vi "TVC_PAT.vi"() -> ()   [LabVIEW 2019]
uses:
  <vilib>/Utility/error.llb/DialogType.ctl
  <vilib>/DAQmx/read.llb/DAQmx Read (Analog 1D DBL NChan 1Samp).vi
  <vilib>/DAQmx/create/channels.llb/DAQmx Create Channel (AI-Voltage-Basic).vi
  <vilib>/DAQmx/configure/timing.llb/DAQmx Timing (Sample Clock).vi
  <vilib>/DAQmx/miscellaneous.llb/DAQmx Fill In Error Info.vi
panel:
  out "THETA ANGLE":dbl(knob) scale=-45.0..45.0
  out "PHI ANGLE":dbl(knob) scale=-45.0..45.0
  in  "Testing Name":string="Postion Accuracy Test"
  in  "File Path":path=path "C:/Users/Kaylin Gopal/Desktop/TVC_electronics/PAT1.tdms"
  in  "?":bool
  in  "Y-Axis":tag
  in  "X-Axis":tag
  # "Channel Settings"
  # "Team: Thrust Vector Control\nTest: Position Accuracy \nAuthour: Kaylin Gopal\n\nPurpose:\n\nDetermine the vectoring accuraccy of the \nthrust vector control test stand."
  # "Equipment:\n\n1. Ultramotion A2 actuators (P - controller)\n2. TE dual axis inclinometer\n3. TVC test stand"
  # "File Settings"
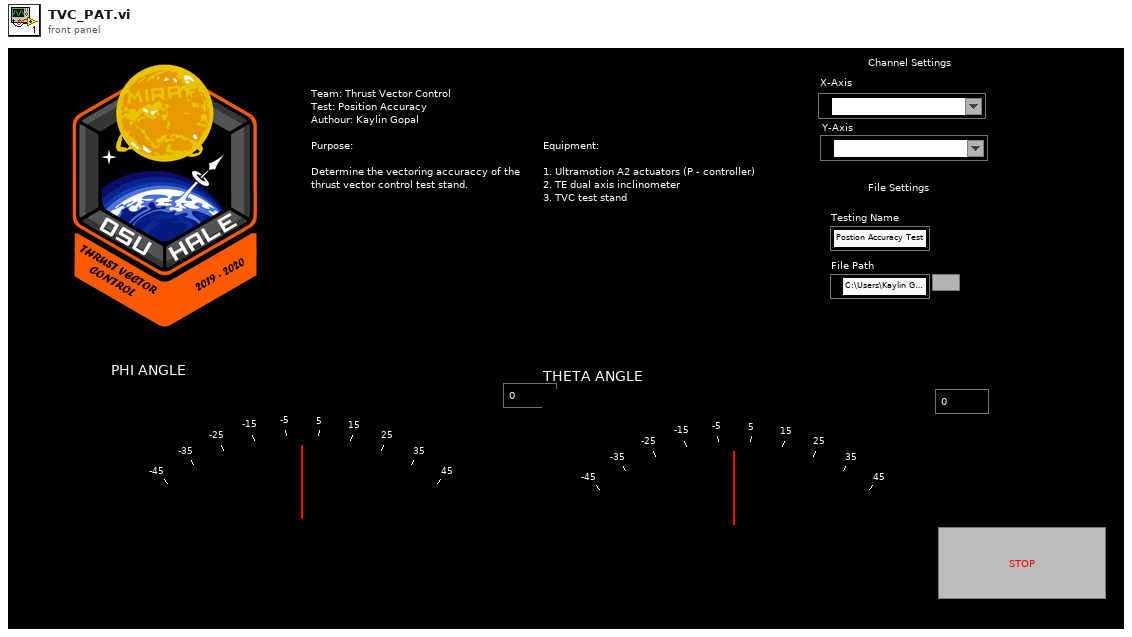
[diagram p1: front panel]
types:
  T1 = typedef "DialogType.ctl" = u16
  T2 = enum16{"open", "open or create", "create or replace", "create", "open (read-only)"}
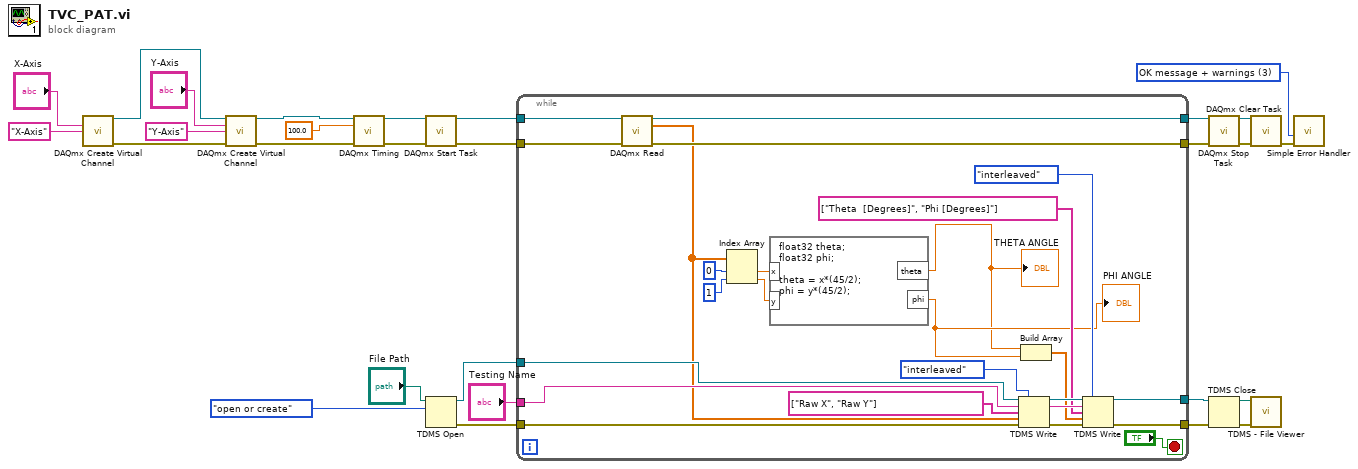
[diagram p0: block diagram]
diagram:
  w3 = T1 3 items=["no dialog", "OK message", "continue or stop message", "OK message + warnings", "continue/stop + warnings"] ("type of dialog (OK msg:1)")
  n1 = call-poly <vilib>:"DAQmx Create Virtual Channel.vi"("physical channels"="X-Axis", "name to assign"="X-Axis") -> ("task out"=w28:refnum<k21>, "error out"=w27:errorcluster)  [unwired: 12 in]
  n2 = call-poly <vilib>:"DAQmx Create Virtual Channel.vi"("task in"=w28, "physical channels"="Y-Axis", "name to assign"="Y-Axis", "error in"=w27) -> ("task out"=w21:refnum<k21>, "error out"=w22:errorcluster)  [unwired: 10 in]
  n3 = call-poly <vilib>:"DAQmx Timing.vi"("task/channels in"=w21, "rate"=100.0, "error in"=w22) -> ("task out"=w18:refnum<k21>, "error out"=w19:errorcluster)  [unwired: 11 in]
  n4 = call <vilib>:"DAQmx Start Task.vi"("task/channels in"=w18, "error in"=w19) -> ("task out"=w16:refnum<k21>, "error out"=w17:errorcluster)  [unwired: 12 in]
  n5 = TDMS Open(10:T2."open or create" ("operation (0:open)"), 11:"File Path") -> (0:w14:errorcluster, 3:w15:refnum<k34>)  [unwired: 5 in]
  n6 = while {
    tunnel: w17 -> [w49]
    tunnel: w16 -> [w48]
    tunnel: w15 -> [w52]
    tunnel: w14 -> [w51]
    tunnel: "Testing Name" -> [w50]
    tunnel: [w40] -> w10
    tunnel: [w39] -> w9
    tunnel: [w45] -> w8
    tunnel: [w44] -> w7
    stop <- "?" stop-if-true
    n7 = call-poly <vilib>:"DAQmx Read.vi"("task/channels in"=w48, "error in"=w49) -> ("task out"=w45:refnum<k21>, "data"=w32:dbl[], "error out"=w44:errorcluster)  [unwired: 11 in]
    n8 = Index Array(array=w32, index #1=0 ("index"), index #2=1 ("index")) -> (element #1=w31:dbl, element #2=w36:dbl)
    n9 = formula code="float32 theta;\nfloat32 phi;\n\ntheta = x*(45/2);\nphi = y*(45/2);"("x"=w31, "y"=w36) -> ("theta"=w29:sgl, "phi"=w30:sgl)
    "THETA ANGLE" <- w29
    "PHI ANGLE" <- w30
    n10 = TDMS Write(0:w52, 1:enum16{"decimated", "interleaved"}."interleaved" ("data layout (0:decimated)"), 5:w50, 7:string[] ["Raw X", "Raw Y"] ("channel name(s) in (Untitled)"), 9:w32, 11:w51) -> (4:w43:refnum<k34>, 6:w41:string, 15:w42:errorcluster)  [unwired: 1 out]
    n11 = Build Array(w29, w30) -> (w34:sgl[])
    n12 = TDMS Write(0:w43, 1:enum16{"decimated", "interleaved"}."interleaved" ("data layout (0:decimated)"), 5:w41, 7:string[] ["Theta  [Degrees]", "Phi [Degrees]"] ("channel name(s) in (Untitled)"), 9:w34, 11:w42) -> (4:w40:refnum<k34>, 15:w39:errorcluster)  [unwired: 2 out]
  }
  n13 = call <vilib>:"DAQmx Stop Task.vi"("task/channels in"=w8, "error in"=w7) -> ("task out"=w6:refnum<k21>, "error out"=w5:errorcluster)  [unwired: 12 in]
  n14 = TDMS Close(8:w9, 11:w10) -> (0:w2:errorcluster, 3:w1:path)
  n15 = call <vilib>:"DAQmx Clear Task.vi"("task in"=w6, "error in"=w5) -> ("error out"=w4:errorcluster)  [unwired: 13 in]
  n16 = call <vilib>:"TDMS - File Viewer.vi"("error in (no error)"=w2, "file path"=w1) -> ()  [unwired: 4 in, 2 out]
  n17 = call <vilib>:"Simple Error Handler.vi"("type of dialog (OK msg:1)"=w3, "error in (no error)"=w4) -> ()  [unwired: 3 in, 5 out]
